vi "sedSpectrometer_cancelCallback_logEvent_AppliedSettingsMatchStart.vi"(8 "error in (no error)":errorcluster) -> (0 "error out":errorcluster, 3 "function return":i32)   [LabVIEW 2016, in "SALLV_sedSpectrometer.lvlib"]
doc: "int sedSpectrometer_shm_cancelCallback_logevent_AppliedSettingsMatchStartLV();"
uses:
  SALLV_sedSpectrometer.lvlib
  SALLV_sedSpectrometer.so
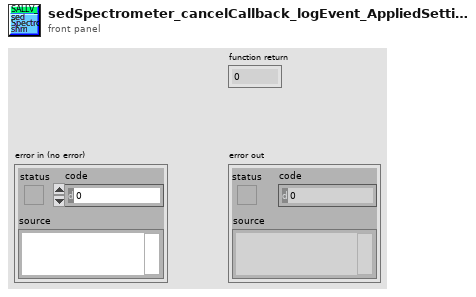
[diagram p1: front panel]
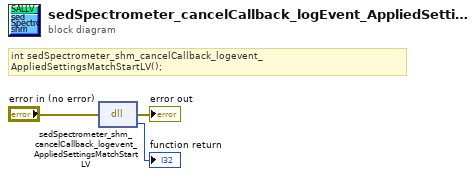
[diagram p0: block diagram]
diagram:
  # "int sedSpectrometer_shm_cancelCallback_logevent_AppliedSettingsMatchStartLV();"
  n1 = dll-call lib="home/harini/TCS/sallv_sedSpectrometer/SALLV_sedSpectrometer.*" fn="sedSpectrometer_shm_cancelCallback_logevent_AppliedSettingsMatchStartLV"(error in="error in (no error)") -> (error out=→"error out":errorcluster, →"function return":i32)  [unwired: 2 in, 1 out]
